vi "Target2.vi"() -> ()   [LabVIEW 2025]
uses:
  <vilib>/Platform/TimedLoop/XDataNode/timing_clust.ctl
  <vilib>/Platform/TimedLoop/XDataNode/nitl_modes.ctl
  <vilib>/Platform/TimedLoop/XDataNode/wakeup.ctl
  <vilib>/rvi/Emulation/niFpgaSctlEmulationGetInTimedLoop.vi
  <vilib>/rvi/Emulation/niFpgaEmulationReportErrorSimple.vi
  <vilib>/rvi/Emulation/niFpgaGetClockAttributes.vi
  <vilib>/rvi/Emulation/niFpgaCriticalErrorInLSC.vi
  <vilib>/rvi/linearAlgebra/MatrixMultiply/simVIs/SubVI/nifxpla_MatrixMultiply_SimMatrixSizes.vi
  <vilib>/rvi/linearAlgebra/MatrixMultiply/simVIs/SubVI/nifxpla_MatrixMultiply_Sim4WireAdapterVector.vi
  <vilib>/rvi/linearAlgebra/MatrixMultiply/simVIs/SubVI/nifxpla_MatrixMultiply_SimFrameHandShake.vi
  <vilib>/rvi/linearAlgebra/MatrixMultiply/simVIs/SubVI/nifxpla_MatrixMultiply_SimEndlessCounter.vi
  <vilib>/rvi/linearAlgebra/MatrixMultiply/simVIs/SubVI/nifxpla_MatrixMultiply_SimVectorDataBuffer.vi
  <vilib>/rvi/ClientSDK/Core/DevComputerLib/Private/Multiply(dfxp64).vi
  <vilib>/rvi/ClientSDK/Core/DevComputerLib/Private/Dfxp128ToDfxp256.vi
  <vilib>/rvi/ClientSDK/Core/DevComputerLib/Private/Add(dfxp256).vi
  <vilib>/rvi/ClientSDK/Core/DevComputerLib/Private/Subtract(dfxp256).vi
  <vilib>/rvi/ClientSDK/Core/DevComputerLib/Private/ToDfxp64(dfxp256).vi
  <vilib>/platform/TimedLoop/XDataNode/XDataNode.xnode
  <vilib>/rvi/linearAlgebra/MatrixMultiply/XNode/nifxpla_MatrixMultiply.xnode
  <vilib>/rvi/linearAlgebra/MatrixMultiply/simVIs/nifxpla_MatrixMultiply_SimTemplateEinEout.vi
  <vilib>/rvi/linearAlgebra/MatrixMultiply/simVIs/nifxpla_MatrixMultiply_SimTemplateEinVout.vi
  <vilib>/rvi/linearAlgebra/MatrixMultiply/simVIs/nifxpla_MatrixMultiply_SimTemplateVinEout.vi
  <vilib>/rvi/linearAlgebra/MatrixMultiply/simVIs/nifxpla_MatrixMultiply_SimTemplateVinVout.vi
  <vilib>/Platform/TimedLoop/XDataNode/XDNodeRunTimeDep.lvlib
panel:
  out "cr 2":fxp<+/-,32,16>[](array[numeric])
  out "appended array":fxp<+/-,32,16>[](array[numeric])
  out "appended array 2":fxp<+/-,32,16>[](array[numeric])
  out "element":fxp<+/-,32,16>
  out "element 2":fxp<+/-,32,16>
  out "element 3":fxp<+/-,32,16>
  out "element 4":fxp<+/-,32,16>
  out "cr":fxp<+/-,32,16>[](array[numeric])
  out "Numeric":i32
  out "Case Number":i16
  out "interleaved array":fxp<+/-,32,16>[](array[numeric])
  out "interleaved array 2":fxp<+/-,32,16>[](array[numeric])
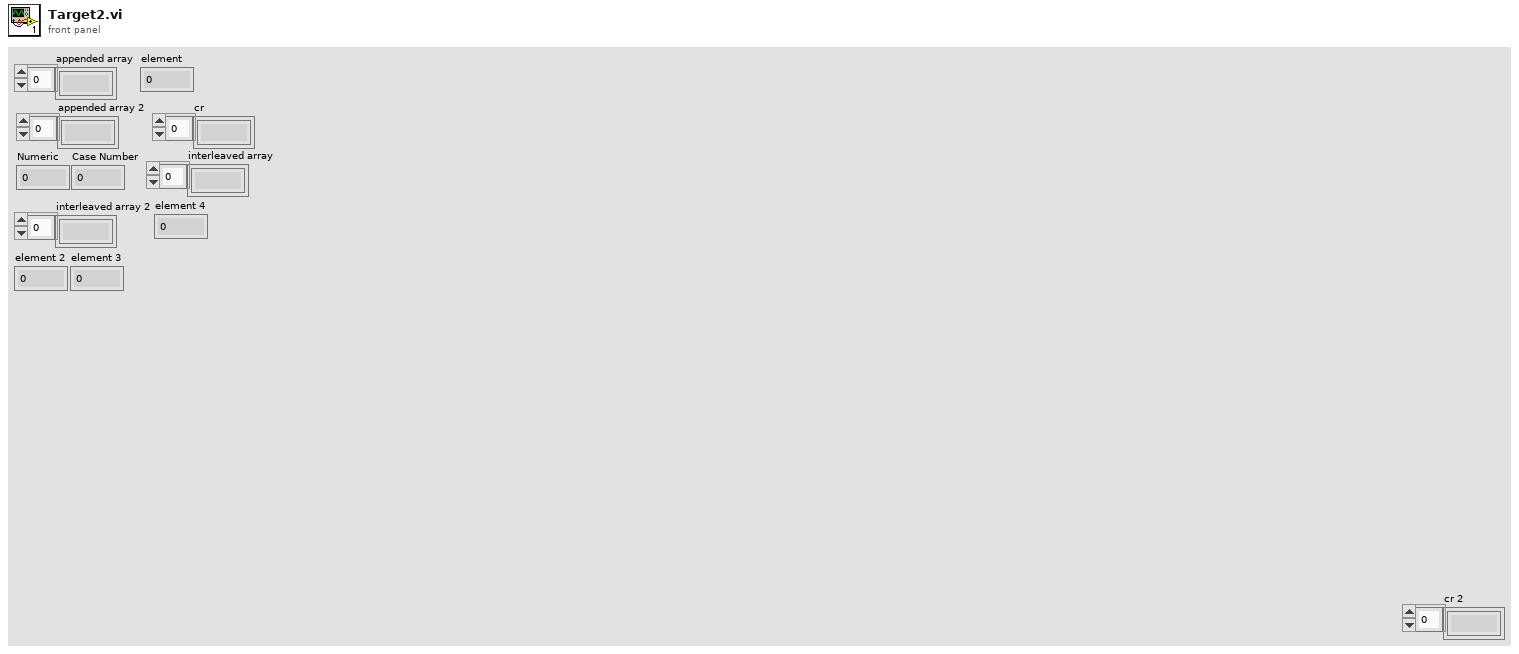
[diagram p1: front panel]
types:
  T1 = typedef "XDNodeRunTimeDep.lvlib/timing_clust.ctl" = cluster{"Expected End [f-1]":u64, "Actual End [f-1]":u64, "Finished Late? [f-1]":bool, "Expected End [i-1]":u64, "Actual End [i-1]":u64, "Finished Late? [i-1]":bool, "Expected Start [i]":u64, "Actual Start [i]":u64, "Expected Start [f]":u64, "Actual Start [f]":u64, "Source Name":string, "Structure Name":string, "Period":i64, "Deadline":i64, "Offset":i64, "Start":i64, "Priority":i32, "Timeout":i32, "Mode":T2, "Wakeup Reason":T3, "Error":errorcluster, "Source Type":string, "Secondary Source Type":string, "Global End Time":u64, "Global Start Time":u64, "Frame Duration":u64, "Iteration Duration":u64, "Assigned CPU":i32, "I/O Scan Engine Mode":u32}
  T2 = typedef "XDNodeRunTimeDep.lvlib/nitl_modes.ctl" = enum32{"No Change", "Process missed periods, maintain original phase", "Discard missed periods, maintain original phase", "Process missed periods, ignore original phase", "Discard missed periods, ignore original phase"}
  T3 = typedef "XDNodeRunTimeDep.lvlib/wakeup.ctl" = enum32{"Normal", "Aborted", "Asynchronous wakeup", "Timing source error", "Timed loop error", "Timeout"}
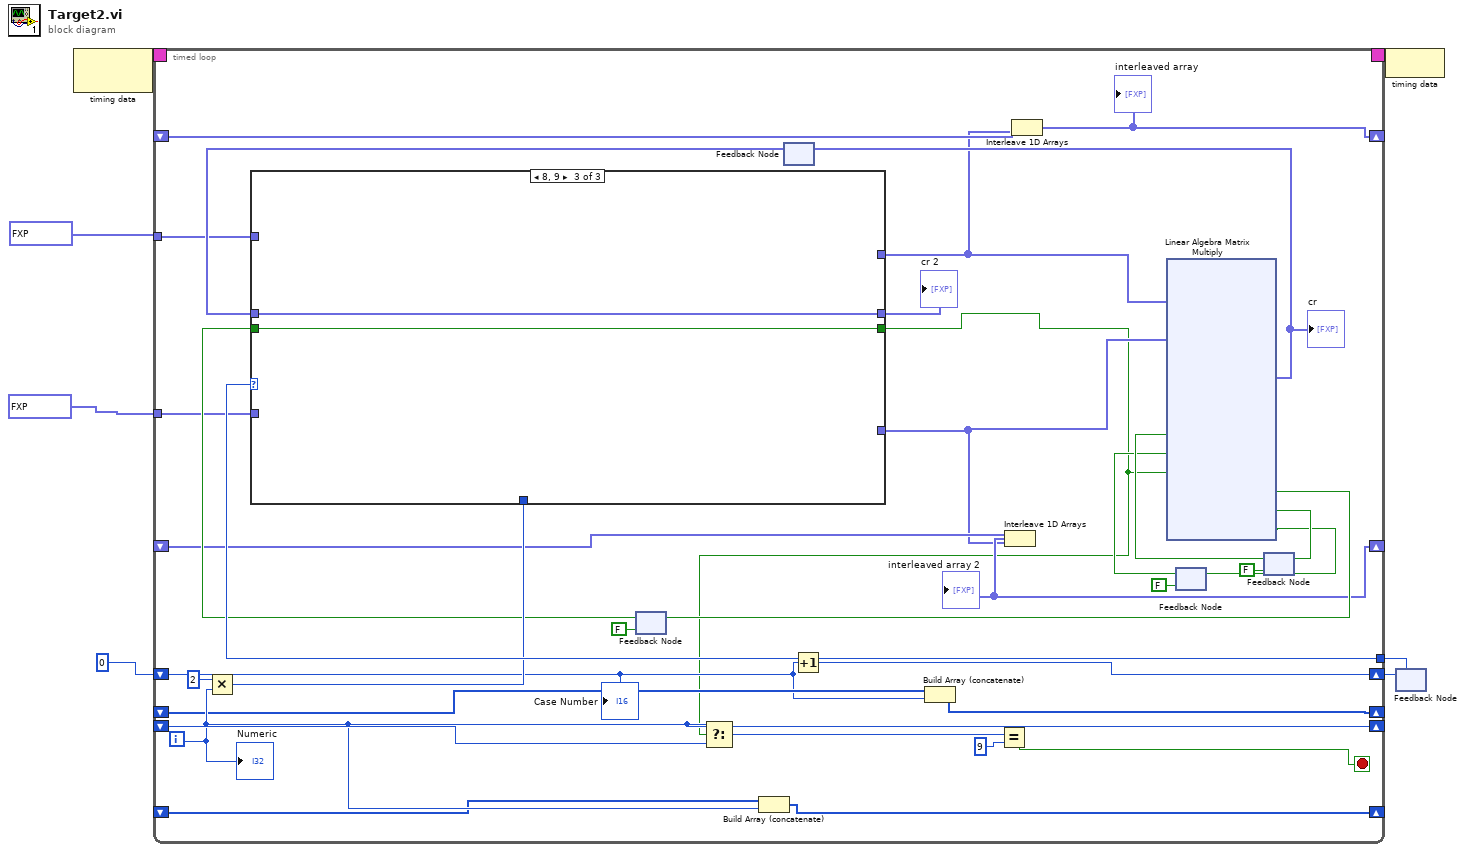
[diagram p0: block diagram]
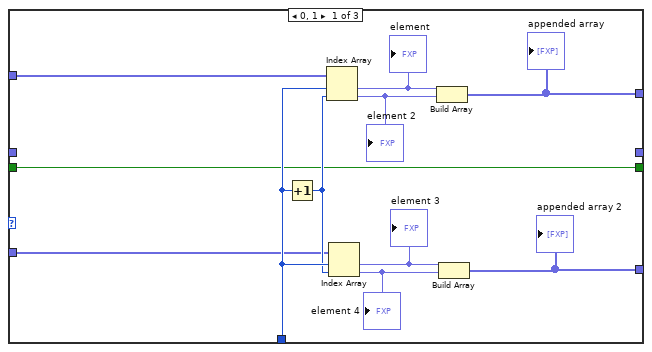
[diagram p2: hidden frame]
diagram:
  n1 = node-c288() -> (w7:T1)  [unwired: 1 in]
  n2 = feedback #1() -> (w3:i16)  [unwired: 1 in]
  n3 = timed-loop {
    timing: w7 -> [_]
    timing-out: [_] -> w6
    shift-right: [w42] -> w4
    shift-left: i16 0 -> [w9]
    tunnel: w3 -> [w41]
    shift-right: [w14] -> _
    shift-left: _ -> [w30]
    tunnel: fxp<+,1,1>[] [1.0, 1.0] -> [w23]
    tunnel: fxp<+,1,2>[] [2.0, 2.0] -> [w22]
    shift-right: [w18] -> _
    shift-left: _ -> [w19]
    shift-right: [w17] -> _
    shift-left: _ -> [w20]
    shift-right: [w12] -> _
    shift-left: _ -> [w13]
    shift-right: [w10] -> _
    shift-left: _ -> [w11]
    i -> [w14]
    stop <- w27 stop-if-true
    n4 = Multiply(x=2, y=w14) -> (x*y=w39:i32)
    n5 = feedback #2(FALSE ("output valid")) -> (w25:bool)
    n6 = Build Array (concatenate)(w13, w14) -> (w12:i32[])
    n7 = feedback #3() -> (w37:fxp<+/-,32,16>[])  [unwired: 1 in]
    n8 = case shown="8, 9" w41 {
      tunnel: [w49 _ _] -> w16
      tunnel: [w48 _ _] -> w15
      tunnel: w39 -> [w47 _ _]
      tunnel: w37 -> [_ _ w56]
      tunnel: w25 -> [w43 w54 w55]
      tunnel: w23 -> [w45 _ _]
      tunnel: w22 -> [w44 _ _]
      tunnel: [_ _ w56] -> w21
      tunnel: [w43 w54 w55] -> w8
      frame 0, 1 {
        n9 = Increment(x=w47) -> (x+1=w46:i32)
        n10 = Index Array(array=w45, index #1=w47, index #2=w46) -> (element #1=w51:fxp<+,1,1>, element #2=w50:fxp<+,1,1>)
        "element" <- w51
        "element 2" <- w50
        n11 = Index Array(array=w44, index #1=w47, index #2=w46) -> (element #1=w53:fxp<+,1,2>, element #2=w52:fxp<+,1,2>)
        "element 3" <- w53
        "element 4" <- w52
        n12 = Build Array(w51, w50) -> (w49:fxp<+,1,1>[])
        "appended array" <- w49
        n13 = Build Array(w53, w52) -> (w48:fxp<+,1,2>[])
        "appended array 2" <- w48
      }
      frame 2, Default {
      }
      frame 8, 9 {
      }
    }
    "cr 2" <- w21
    n14 = Select(t=w14, s=w8, f=w30) -> (s? t:f=w29:i32)
    n15 = Increment(x=w9) -> (x+1=w42:i16)
    n16 = Build Array (concatenate)(w11, w9) -> (w10:i16[])
    n17 = Equal?(x=w29, y=9) -> (x = y?=w27:bool)
    n18 = Interleave 1D Arrays(w20, w15) -> (w17:fxp<+,1,2>[])
    "interleaved array 2" <- w17
    n19 = Interleave 1D Arrays(w19, w16) -> (w18:fxp<+,1,1>[])
    "interleaved array" <- w18
    n20 = feedback #4(FALSE ("ready for b")) -> (w33:bool)
    n21 = feedback #5(FALSE ("ready for a")) -> (w35:bool)
    n22 = xnode ("Linear Algebra Matrix Multiply")("ar"=w16, "br"=w15, "a valid"=w35, "b valid"=w33, "ready for output (T)"=w8) -> ("cr"=w38:fxp<+/-,32,16>[], "output valid"=w26:bool, "ready for a"=w36:bool, "ready for b"=w34:bool)  [unwired: 2 in, 2 out]
    "cr" <- w38
    n23 = feedback-in #2(w26) -> ()
    n24 = feedback-in #3(w38) -> ()
    n25 = feedback-in #4(w34) -> ()
    n26 = feedback-in #5(w36) -> ()
    "Numeric" <- w14
    "Case Number" <- w9
  }
  n27 = node-c288(w6) -> ()
  n28 = feedback-in #1(w4) -> ()
